vi "Lookup API.vi"(8 "error in (no error)":errorcluster, 9 "Promise":refnum<class "Promise.lvclass">, 10 "Identity":refnum<class "Identity.lvclass">, 11 "VolatusCore in":refnum<class "VolatusCore.lvclass">) -> (0 "error out":errorcluster, 3 "VolatusCore out":refnum<class "VolatusCore.lvclass">)   [LabVIEW 2020, in "Volatus.lvlib" / "VolatusCore.lvclass"]
uses:
  VolatusCore.lvclass
  Identity/Identity.lvclass
  VolatusCore.lvclass/VolatusCore.ctl
  ApiValue/ApiValue.lvclass
  lv-promises/Promises/Promise/Promise.lvclass
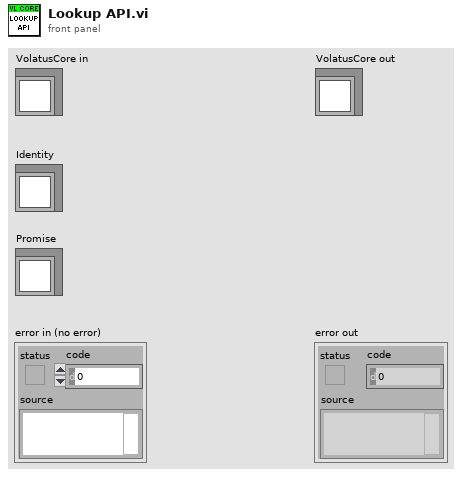
[diagram p1: front panel]
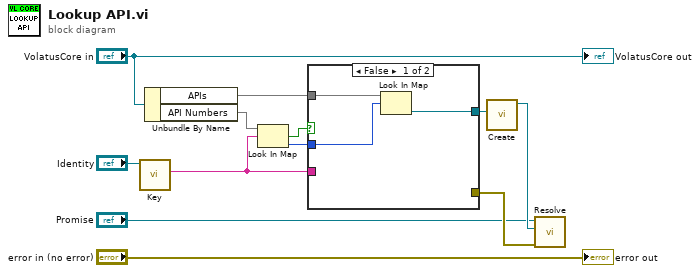
[diagram p0: block diagram]
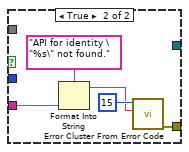
[diagram p2: hidden frame]
diagram:
  n1 = call "Key.vi"("Identity in"="Identity") -> ("Key"=w5:string)  [unwired: 10 in]
  n2 = Unbundle By Name("VolatusCore in") -> ("APIs"=w7:map{u32, refnum<class "API.lvclass">}, "API Numbers"=w9:map{string, u32})
  n3 = Look In Map(map=w9, key=w5) -> (key not found?=w8:bool, value=w6:u32)  [unwired: 1 in]
  n4 = case shown="False" w8 {
    tunnel: w7 -> [w15 _]
    tunnel: w6 -> [w14 _]
    tunnel: w5 -> [_ w19]
    tunnel: [w13 _] -> w4
    tunnel: [_ w16] -> w3
    frame False {
      n5 = Look In Map(map=w15, key=w14) -> (value=w13:refnum<class "API.lvclass">)  [unwired: 1 in, 1 out]
    }
    frame True {
      n6 = Format Into String(format string="API for identity \"%s\" not found.", w19) -> (resulting string=w17:string)  [unwired: 2 in, 1 out]
      n7 = call <vilib>:"Error Cluster From Error Code.vi"("error message (\"\")"=w17, "error code (0)"=15) -> ("error out"=w16:errorcluster)  [unwired: 7 in]
    }
  }
  n8 = call "Create.vi"("API"=w4) -> ("ApiValue out"=w2:refnum<class "ApiValue.lvclass">)  [unwired: 10 in]
  n9 = call "Resolve.vi"("error in (no error)"=w3, "Result"=w2, "Promise in"="Promise") -> ()  [unwired: 7 in, 2 out]
  "error out" <- "error in (no error)"
  "VolatusCore out" <- "VolatusCore in"
